vi "8 PulseMeasurements.vi"(2 "8 PulseMeas Chs":T1={"DI0"="Connector0/DIO0", "DI1"="Connector0/DIO1", "DI2"="Connector0/DIO2", "DI3"="Connector0/DIO3", "DI4"="Connector0/DIO8", "DI5"="Connector0/DIO9", "DI6"="Connector0/DIO10", "DI7"="Connector0/DIO11"}, 4 "PulseMeas Timeouts":u32[](array[numeric])=[0, 0, 0, 0, 0, 0, 0, 0]) -> (7 "PulseMeas Packets":u64[](array[numeric]))   [LabVIEW 2010]
uses:
  <vilib>/eio/EIONode/EIONode.xnode
  <vilib>/rvi/eio/nirviEIOImplementation/nirviEIOImplementation.xnode
  <vilib>/rvi/eio/common/nirviEmuClasses.ctl
  <vilib>/rvi/eio/common/nirviEmuTemplateMethod_noerrors.vi
  <vilib>/NI Veristand/FPGA/NI_VS FPGA Support.lvlib
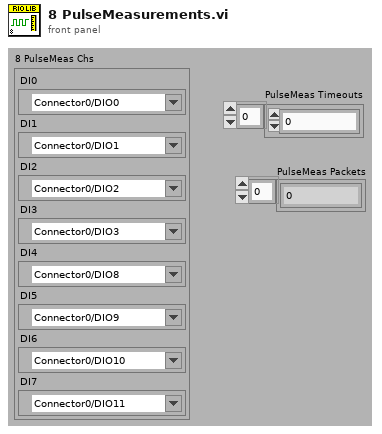
[diagram p1: front panel]
types:
  T1 = cluster{"DI0":refnum<k21>, "DI1":refnum<k21>, "DI2":refnum<k21>, "DI3":refnum<k21>, "DI4":refnum<k21>, "DI5":refnum<k21>, "DI6":refnum<k21>, "DI7":refnum<k21>}
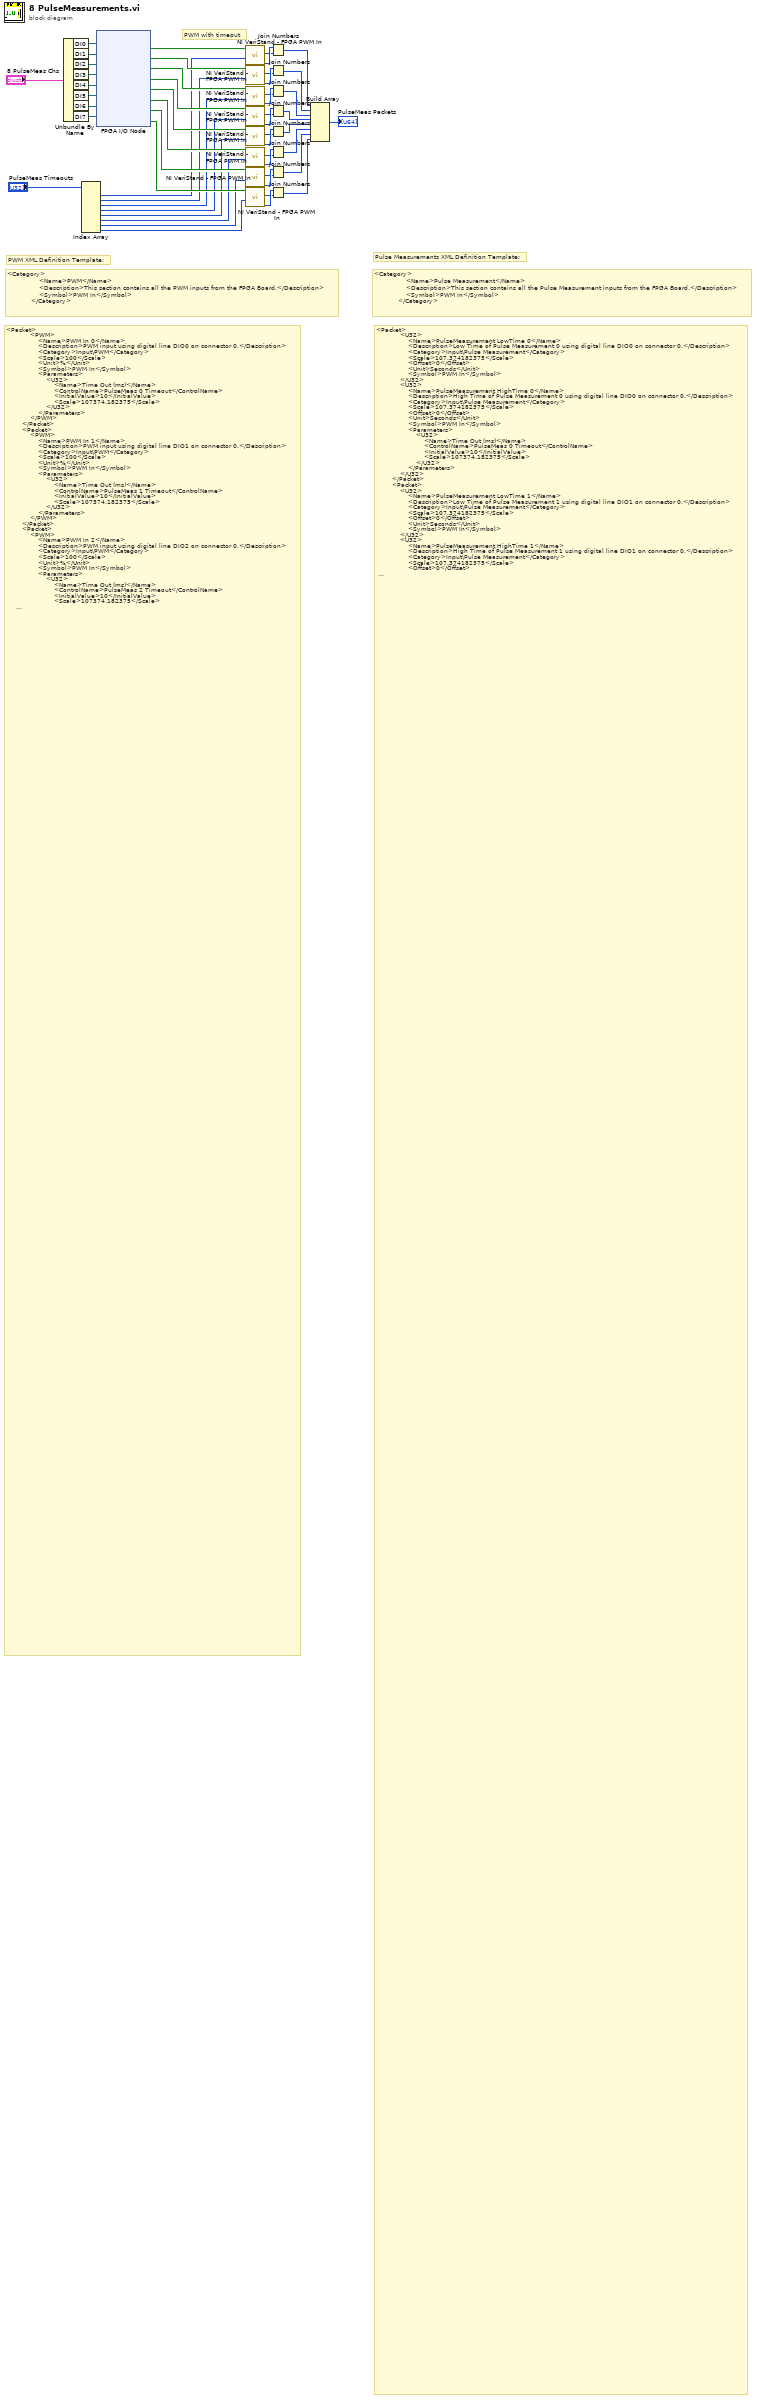
[diagram p0: block diagram]
diagram:
  # "<Category>\n                <Name>PWM</Name>\n                <Description>This section contains all the PWM inputs from the FPGA Board.</Description>\n                <Symbol>PWM In</Symbol>\n            </Category>"
  # "<Category>\n                <Name>Pulse Measurement</Name>\n                <Description>This section contains all the Pulse Measurement inputs from the FPGA Board.</Description>\n                <Symbol>PWM In</Symbol>\n            </Category>"
  # "Pulse Measurements XML Definition Template:"
  # "<Packet>\n            <U32>\n                <Name>PulseMeasurement LowTime 0</Name>\n                <Description>Low Time of Pulse Measurement 0 using digital line DIO0 on connector 0.</Description>\n                <Category>Input\\Pulse Measurement</Category>\n                <Scale>107.374182375</Scale>\n                <Offset>0</Offset>\n                <Unit>Seconds</Unit>\n                <Symbol>PWM In</Symbol>\n            </U32>\n            <U32>\n                <Name>PulseMeasurement HighTime 0</Name>\n                <Description>High Time of Pulse Measurement 0 using digital line DIO0 on connector 0.</Description>\n                <Category>Input\\Pulse Measurement</Category>\n                <Scale>107.374182375</Scale>\n                <Offset>0</Offset>\n                <Unit>Seconds</Unit>\n                <Symbol>PWM In</Symbol>\n                <Parameters>\n                    <U32>\n                        <Name>Time Out (ms)</Name>\n                        <ControlName>PulseMeas 0 Timeout</ControlName>\n                        <InitialValue>10</InitialValue>\n                        <Scale>107374.182375</Scale>\n                    </U32>\n                </Parameters>\n            </U32>\n        </Packet>\n        <Packet>\n            <U32>\n                <Name>PulseMeasurement LowTime 1</Name>\n                <Description>Low Time of Pulse Measurement 1 using digital line DIO1 on connector 0.</Description>\n                <Category>Input\\Pulse Measurement</Category>\n                <Scale>107.374182375</Scale>\n                <Offset>0</Offset>\n                <Unit>Seconds</Unit>\n                <Symbol>PWM In</Symbol>\n            </U32>\n            <U32>\n                <Name>PulseMeasurement HighTime 1</Name>\n                <Description>High Time of Pulse Measurement 1 using digital line DIO1 on connector 0.</Description>\n                <Category>Input\\Pulse Measurement</Category>\n                <Scale>107.374182375</Scale>\n                <Offset>0</Offset>\n                <Unit>Seconds</Unit>\n                <Symbol>PWM In</Symbol>\n                <Parameters>\n                    <U32>\n                        <Name>Time Out (ms)</Name>\n                        <ControlName>PulseMeas 1 Timeout</ControlName>\n                        <InitialValue>10</InitialValue>\n                        <Scale>107374.182375</Scale>\n                    </U32>\n                </Parameters>\n            </U32>\n        </Packet>\n        <Packet>\n            <U32>\n                <Name>PulseMeasurement LowTime 2</Name>\n                <Description>Low Time of Pulse Measurement 2 using digital line DIO2 on connector 0.</Description>\n                <Category>Input\\Pulse Measurement</Category>\n                <Scale>107.374182375</Scale>\n                <Offset>0</Offset>\n                <Unit>Seconds</Unit>\n                <Symbol>PWM In</Symbol>\n            </U32>\n            <U32>\n                <Name>PulseMeasurement HighTime 2</Name>\n                <Description>High Time of Pulse Measurement 2 using digital line DIO2 on connector 0.</Description>\n                <Category>Input\\Pulse Measurement</Category>\n                <Scale>107.374182375</Scale>\n                <Offset>0</Offset>\n                <Unit>Seconds</Unit>\n                <Symbol>PWM In</Symbol>\n                <Parameters>\n                    <U32>\n                        <Name>Time Out (ms)</Name>\n                        <ControlName>PulseMeas 2 Timeout</ControlName>\n                        <InitialValue>10</InitialValue>\n                        <Scale>107374.182375</Scale>\n                    </U32>\n                </Parameters>\n            </U32>\n        </Packet>\n        <Packet>\n            <U32>\n                <Name>PulseMeasurement LowTime 3</Name>\n                <Description>Low Time of Pulse Measurement 3 using digital line DIO3 on connector 0.</Description>\n                <Category>Input\\Pulse Measurement</Category>\n                <Scale>107.374182375</Scale>\n                <Offset>0</Offset>\n                <Unit>Seconds</Unit>\n                <Symbol>PWM In</Symbol>\n            </U32>\n            <U32>\n                <Name>PulseMeasurement HighTime 3</Name>\n                <Description>High Time of Pulse Measurement 3 using digital line DIO3 on connector 0.</Description>\n                <Category>Input\\Pulse Measurement</Category>\n                <Scale>107.374182375</Scale>\n                <Offset>0</Offset>\n                <Unit>Seconds</Unit>\n                <Symbol>PWM In</Symbol>\n                <Parameters>\n                    <U32>\n                        <Name>Time Out (ms)</Name>\n                        <ControlName>PulseMeas 3 Timeout</ControlName>\n                        <InitialValue>10</InitialValue>\n                        <Scale>107374.182375</Scale>\n                    </U32>\n                </Parameters>\n            </U32>\n        </Packet>\n        <Packet>\n            <U32>\n                <Name>PulseMeasurement LowTime 4</Name>\n                <Description>Low Time of Pulse Measurement 4 using digital line DIO8 on connector 0.</Description>\n                <Category>Input\\Pulse Measurement</Category>\n                <Scale>107.374182375</Scale>\n                <Offset>0</Offset>\n                <Unit>Seconds</Unit>\n                <Symbol>PWM In</Symbol>\n            </U32>\n            <U32>\n                <Name>PulseMeasurement HighTime 4</Name>\n                <Description>High Time of Pulse Measurement 4 using digital line DIO8 on connector 4.</Description>\n                <Category>Input\\Pulse Measurement</Category>\n                <Scale>107.374182375</Scale>\n                <Offset>0</Offset>\n                <Unit>Seconds</Unit>\n                <Symbol>PWM In</Symbol>\n                <Parameters>\n                    <U32>\n                        <Name>Time Out (ms)</Name>\n                        <ControlName>PulseMeas 4 Timeout</ControlName>\n                        <InitialValue>10</InitialValue>\n                        <Scale>107374.182375</Scale>\n                    </U32>\n                </Parameters>\n            </U32>\n        </Packet>\n        <Packet>\n            <U32>\n                <Name>PulseMeasurement LowTime 5</Name>\n                <Description>Low Time of Pulse Measurement 5 using digital line DIO9 on connector 0.</Description>\n                <Category>Input\\Pulse Measurement</Category>\n                <Scale>107.374182375</Scale>\n                <Offset>0</Offset>\n                <Unit>Seconds</Unit>\n                <Symbol>PWM In</Symbol>\n            </U32>\n            <U32>\n                <Name>PulseMeasurement HighTime 5</Name>\n                <Description>High Time of Pulse Measurement 5 using digital line DIO9 on connector 0.</Description>\n                <Category>Input\\Pulse Measurement</Category>\n                <Scale>107.374182375</Scale>\n                <Offset>0</Offset>\n                <Unit>Seconds</Unit>\n                <Symbol>PWM In</Symbol>\n                <Parameters>\n                    <U32>\n                        <Name>Time Out (ms)</Name>\n                        <ControlName>PulseMeas 5 Timeout</ControlName>\n                        <InitialValue>10</InitialValue>\n                        <Scale>107374.182375</Scale>\n                    </U32>\n                </Parameters>\n            </U32>\n        </Packet>\n        <Packet>\n            <U32>\n                <Name>PulseMeasurement LowTime 6</Name>\n                <Description>Low Time of Pulse Measurement 6 using digital line DIO10 on connector 0.</Description>\n                <Category>Input\\Pulse Measurement</Category>\n                <Scale>107.374182375</Scale>\n                <Offset>0</Offset>\n                <Unit>Seconds</Unit>\n                <Symbol>PWM In</Symbol>\n            </U32>\n            <U32>\n                <Name>PulseMeasurement HighTime 6</Name>\n                <Description>High Time of Pulse Measurement 6 using digital line DIO10 on connector 0.</Description>\n                <Category>Input\\Pulse Measurement</Category>\n                <Scale>107.374182375</Scale>\n                <Offset>0</Offset>\n                <Unit>Seconds</Unit>\n                <Symbol>PWM In</Symbol>\n                <Parameters>\n                    <U32>\n                        <Name>Time Out (ms)</Name>\n                        <ControlName>PulseMeas 6 Timeout</ControlName>\n                        <InitialValue>10</InitialValue>\n                        <Scale>107374.182375</Scale>\n                    </U32>\n                </Parameters>\n            </U32>\n        </Packet>\n        <Packet>\n            <U32>\n                <Name>PulseMeasurement LowTime 7</Name>\n                <Description>Low Time of Pulse Measurement 7 using digital line DIO11 on connector 0.</Description>\n                <Category>Input\\Pulse Measurement</Category>\n                <Scale>107.374182375</Scale>\n                <Offset>0</Offset>\n                <Unit>Seconds</Unit>\n                <Symbol>PWM In</Symbol>\n            </U32>\n            <U32>\n                <Name>PulseMeasurement HighTime 7</Name>\n                <Description>High Time of Pulse Measurement 7 using digital line DIO11 on connector 0.</Description>\n                <Category>Input\\Pulse Measurement</Category>\n                <Scale>107.374182375</Scale>\n                <Offset>0</Offset>\n                <Unit>Seconds</Unit>\n                <Symbol>PWM In</Symbol>\n                <Parameters>\n                    <U32>\n                        <Name>Time Out (ms)</Name>\n                        <ControlName>PulseMeas 7 Timeout</ControlName>\n                        <InitialValue>10</InitialValue>\n                        <Scale>107374.182375</Scale>\n                    </U32>\n                </Parameters>\n            </U32>\n        </Packet>"
  # "PWM XML Definition Template:"
  # "<Packet>\n            <PWM>\n                <Name>PWM In 0</Name>\n                <Description>PWM input using digital line DIO0 on connector 0.</Description>\n                <Category>Input\\PWM</Category>\n                <Scale>100</Scale>\n                <Unit>%</Unit>\n                <Symbol>PWM In</Symbol>\n                <Parameters>\n                    <U32>\n                        <Name>Time Out (ms)</Name>\n                        <ControlName>PulseMeas 0 Timeout</ControlName>\n                        <InitialValue>10</InitialValue>\n                        <Scale>107374.182375</Scale>\n                    </U32>\n                </Parameters>\n            </PWM>\n        </Packet>\n        <Packet>\n            <PWM>\n                <Name>PWM In 1</Name>\n                <Description>PWM input using digital line DIO1 on connector 0.</Description>\n                <Category>Input\\PWM</Category>\n                <Scale>100</Scale>\n                <Unit>%</Unit>\n                <Symbol>PWM In</Symbol>\n                <Parameters>\n                    <U32>\n                        <Name>Time Out (ms)</Name>\n                        <ControlName>PulseMeas 1 Timeout</ControlName>\n                        <InitialValue>10</InitialValue>\n                        <Scale>107374.182375</Scale>\n                    </U32>\n                </Parameters>\n            </PWM>\n        </Packet>\n        <Packet>\n            <PWM>\n                <Name>PWM In 2</Name>\n                <Description>PWM input using digital line DIO2 on connector 0.</Description>\n                <Category>Input\\PWM</Category>\n                <Scale>100</Scale>\n                <Unit>%</Unit>\n                <Symbol>PWM In</Symbol>\n                <Parameters>\n                    <U32>\n                        <Name>Time Out (ms)</Name>\n                        <ControlName>PulseMeas 2 Timeout</ControlName>\n                        <InitialValue>10</InitialValue>\n                        <Scale>107374.182375</Scale>\n                    </U32>\n                </Parameters>\n            </PWM>\n        </Packet>\n        <Packet>\n            <PWM>\n                <Name>PWM In 3</Name>\n                <Description>PWM input using digital line DIO3 on connector 0.</Description>\n                <Category>Input\\PWM</Category>\n                <Scale>100</Scale>\n                <Unit>%</Unit>\n                <Symbol>PWM In</Symbol>\n                <Parameters>\n                    <U32>\n                        <Name>Time Out (ms)</Name>\n                        <ControlName>PulseMeas 3 Timeout</ControlName>\n                        <InitialValue>10</InitialValue>\n                        <Scale>107374.182375</Scale>\n                    </U32>\n                </Parameters>\n            </PWM>\n        </Packet>\n        <Packet>\n            <PWM>\n                <Name>PWM In 4</Name>\n                <Description>PWM input using digital line DIO8 on connector 0.</Description>\n                <Category>Input\\PWM</Category>\n                <Scale>100</Scale>\n                <Unit>%</Unit>\n                <Symbol>PWM In</Symbol>\n                <Parameters>\n                    <U32>\n                        <Name>Time Out (ms)</Name>\n                        <ControlName>PulseMeas 4 Timeout</ControlName>\n                        <InitialValue>10</InitialValue>\n                        <Scale>107374.182375</Scale>\n                    </U32>\n                </Parameters>\n            </PWM>\n        </Packet>\n        <Packet>\n            <PWM>\n                <Name>PWM In 5</Name>\n                <Description>PWM input using digital line DIO9 on connector 0.</Description>\n                <Category>Input\\PWM</Category>\n                <Scale>100</Scale>\n                <Unit>%</Unit>\n                <Symbol>PWM In</Symbol>\n                <Parameters>\n                    <U32>\n                        <Name>Time Out (ms)</Name>\n                        <ControlName>PulseMeas 5 Timeout</ControlName>\n                        <InitialValue>10</InitialValue>\n                        <Scale>107374.182375</Scale>\n                    </U32>\n                </Parameters>\n            </PWM>\n        </Packet>\n        <Packet>\n            <PWM>\n                <Name>PWM In 6</Name>\n                <Description>PWM input using digital line DIO10 on connector 0.</Description>\n                <Category>Input\\PWM</Category>\n                <Scale>100</Scale>\n                <Unit>%</Unit>\n                <Symbol>PWM In</Symbol>\n                <Parameters>\n                    <U32>\n                        <Name>Time Out (ms)</Name>\n                        <ControlName>PulseMeas 6 Timeout</ControlName>\n                        <InitialValue>10</InitialValue>\n                        <Scale>107374.182375</Scale>\n                    </U32>\n                </Parameters>\n            </PWM>\n        </Packet>\n        <Packet>\n            <PWM>\n                <Name>PWM In 7</Name>\n                <Description>PWM input using digital line DIO11 on connector 0.</Description>\n                <Category>Input\\PWM</Category>\n                <Scale>100</Scale>\n                <Unit>%</Unit>\n                <Symbol>PWM In</Symbol>\n                <Parameters>\n                    <U32>\n                        <Name>Time Out (ms)</Name>\n                        <ControlName>PulseMeas 8 Timeout</ControlName>\n                        <InitialValue>10</InitialValue>\n                        <Scale>107374.182375</Scale>\n                    </U32>\n                </Parameters>\n            </PWM>\n        </Packet>"
  # "PWM with timeout"
  n1 = Unbundle By Name("8 PulseMeas Chs") -> ("DI0"=w1:refnum<k21>, "DI1"=w2:refnum<k21>, "DI2"=w3:refnum<k21>, "DI3"=w4:refnum<k21>, "DI4"=w5:refnum<k21>, "DI5"=w6:refnum<k21>, "DI6"=w7:refnum<k21>, "DI7"=w8:refnum<k21>)
  n2 = Index Array(array="PulseMeas Timeouts") -> (element #1=w10:u32, element #2=w11:u32, element #3=w12:u32, element #4=w13:u32, element #5=w14:u32, element #6=w15:u32, element #7=w16:u32, element #8=w17:u32)  [unwired: 8 in]
  n3 = xnode "FPGA I/O Node"("FPGA I/O In"=w1, "FPGA I/O In"=w2, "FPGA I/O In"=w3, "FPGA I/O In"=w4, "FPGA I/O In"=w5, "FPGA I/O In"=w6, "FPGA I/O In"=w7, "FPGA I/O In"=w8) -> ("I/O Item"=w19:bool, "I/O Item"=w22:bool, "I/O Item"=w23:bool, "I/O Item"=w24:bool, "I/O Item"=w25:bool, "I/O Item"=w26:bool, "I/O Item"=w27:bool, "I/O Item"=w28:bool)  [unwired: 8 out]
  n4 = call <vilib>:"NI VeriStand - FPGA PWM In.vi"("Time Out"=w10, "Value"=w19) -> ("High time"=w21:u32, "Low Time"=w20:u32)  [unwired: 8 out]
  n5 = call <vilib>:"NI VeriStand - FPGA PWM In.vi"("Time Out"=w11, "Value"=w22) -> ("High time"=w42:u32, "Low Time"=w29:u32)  [unwired: 8 out]
  n6 = call <vilib>:"NI VeriStand - FPGA PWM In.vi"("Time Out"=w12, "Value"=w23) -> ("High time"=w41:u32, "Low Time"=w30:u32)  [unwired: 8 out]
  n7 = call <vilib>:"NI VeriStand - FPGA PWM In.vi"("Time Out"=w13, "Value"=w24) -> ("High time"=w40:u32, "Low Time"=w31:u32)  [unwired: 8 out]
  n8 = call <vilib>:"NI VeriStand - FPGA PWM In.vi"("Time Out"=w14, "Value"=w25) -> ("High time"=w39:u32, "Low Time"=w32:u32)  [unwired: 8 out]
  n9 = call <vilib>:"NI VeriStand - FPGA PWM In.vi"("Time Out"=w15, "Value"=w26) -> ("High time"=w38:u32, "Low Time"=w33:u32)  [unwired: 8 out]
  n10 = call <vilib>:"NI VeriStand - FPGA PWM In.vi"("Time Out"=w16, "Value"=w27) -> ("High time"=w37:u32, "Low Time"=w34:u32)  [unwired: 8 out]
  n11 = call <vilib>:"NI VeriStand - FPGA PWM In.vi"("Time Out"=w17, "Value"=w28) -> ("High time"=w36:u32, "Low Time"=w35:u32)  [unwired: 8 out]
  n12 = Join Numbers(hi=w21, lo=w20) -> ((hi.lo)=w43:u64)
  n13 = Join Numbers(hi=w42, lo=w29) -> ((hi.lo)=w44:u64)
  n14 = Join Numbers(hi=w41, lo=w30) -> ((hi.lo)=w45:u64)
  n15 = Join Numbers(hi=w40, lo=w31) -> ((hi.lo)=w46:u64)
  n16 = Join Numbers(hi=w39, lo=w32) -> ((hi.lo)=w50:u64)
  n17 = Join Numbers(hi=w38, lo=w33) -> ((hi.lo)=w49:u64)
  n18 = Join Numbers(hi=w37, lo=w34) -> ((hi.lo)=w48:u64)
  n19 = Join Numbers(hi=w36, lo=w35) -> ((hi.lo)=w47:u64)
  n20 = Build Array(w43, w44, w45, w46, w50, w49, w48, w47) -> (→"PulseMeas Packets":u64[])
